vi "JSON FV.vi"(8 "error in":errorcluster, 9 "JSON Scalar in 3":refnum<class "JSON Scalar.lvclass">, 10 "JSON Scalar in 2":refnum<class "JSON Scalar.lvclass">, 11 "JSON Scalar in 1":refnum<class "JSON Scalar.lvclass">) -> (0 "error out":errorcluster, 2 "JSON Object out":refnum<class "JSON Object.lvclass">, 3 "Instante":refnum<class "JSON Object.lvclass">)   [LabVIEW 2015]
uses:
  <vilib>/addons/JSON API/Get Polymorphic/JSON GetSet.lvlib
  <vilib>/addons/JSON API/JSON Object/Set Object Item by name.vi
  <vilib>/addons/JSON API/JSON Object/JSON Object.lvclass
  <vilib>/addons/JSON API/JSON Scalar/Set U32.vi
  <vilib>/addons/JSON API/JSON Scalar/JSON Scalar.lvclass
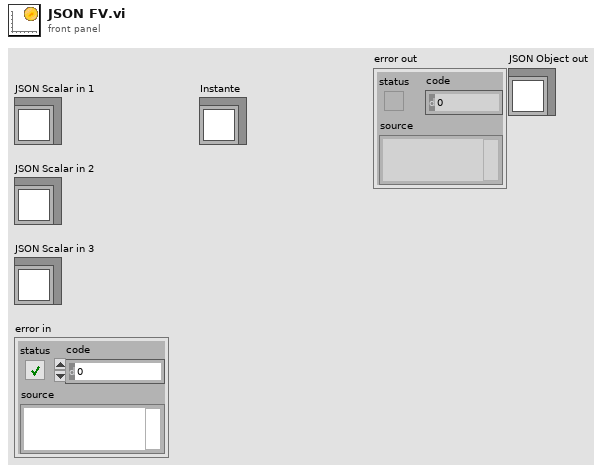
[diagram p1: front panel]
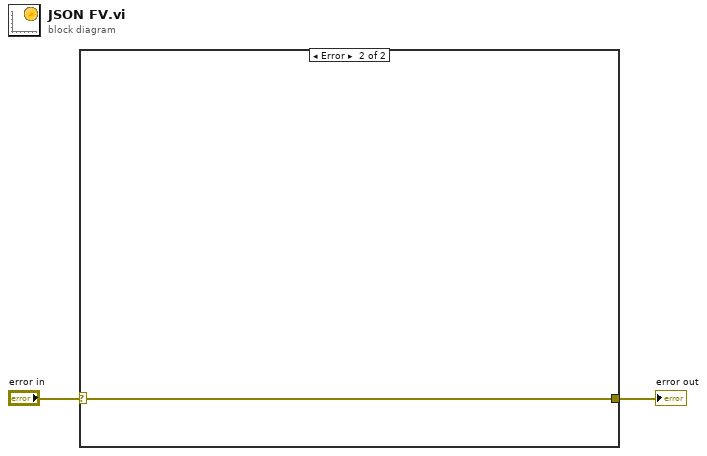
[diagram p0: block diagram]
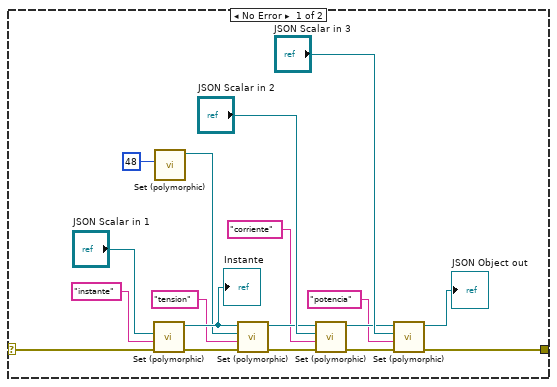
[diagram p2: hidden frame]
diagram:
  n1 = case shown="Error" "error in" {
    selector: "error in" -> [w3 w21]
    tunnel: [w4 w21] -> w2
    frame No Error {
      n2 = call-poly <vilib>:"Set (polymorphic).vi"("error in (no error)"=w3, "name"="instante", "Value"="JSON Scalar in 1") -> ("error out"=w18:errorcluster, "JSON Object out"=w17:refnum<class "JSON Object.lvclass">)  [unwired: 6 in, 1 out]
      "Instante" <- w17
      n3 = call-poly <vilib>:"Set (polymorphic).vi"("Numeric"=u32 48) -> ("JSON Scalar out"=w10:refnum<class "JSON Scalar.lvclass">)  [unwired: 9 in, 1 out]
      n4 = call-poly <vilib>:"Set (polymorphic).vi"("error in (no error)"=w18, "name"="tension", "Value"=w10, "JSON Object in"=w17) -> ("error out"=w19:errorcluster, "JSON Object out"=w11:refnum<class "JSON Object.lvclass">)  [unwired: 5 in, 1 out]
      n5 = call-poly <vilib>:"Set (polymorphic).vi"("error in (no error)"=w19, "name"="corriente", "Value"="JSON Scalar in 2", "JSON Object in"=w11) -> ("error out"=w20:errorcluster, "JSON Object out"=w13:refnum<class "JSON Object.lvclass">)  [unwired: 5 in, 1 out]
      n6 = call-poly <vilib>:"Set (polymorphic).vi"("error in (no error)"=w20, "name"="potencia", "Value"="JSON Scalar in 3", "JSON Object in"=w13) -> ("error out"=w4:errorcluster, "JSON Object out"=→"JSON Object out":refnum<class "JSON Object.lvclass">)  [unwired: 5 in, 1 out]
    }
    frame Error {
    }
  }
  "error out" <- w2
